vi "Read Exception Status Response.vi"(8 "error in (no error)":errorcluster, 10 "Modbus data unit in":refnum<class "Modbus Data Unit (PDU).lvclass">) -> (0 "error out":errorcluster, 2 "exception status":u8)   [LabVIEW 2018, in "SubVIs.lvlib" / "Master Function Definition.lvlib"]
doc: "Decodes the response generated by the read exception status function."
uses:
  Master Function Definition.lvlib
  Modbus Data Unit (PDU).lvclass
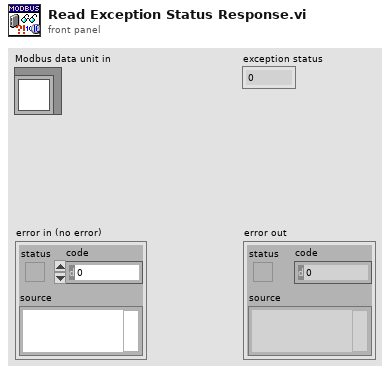
[diagram p1: front panel]
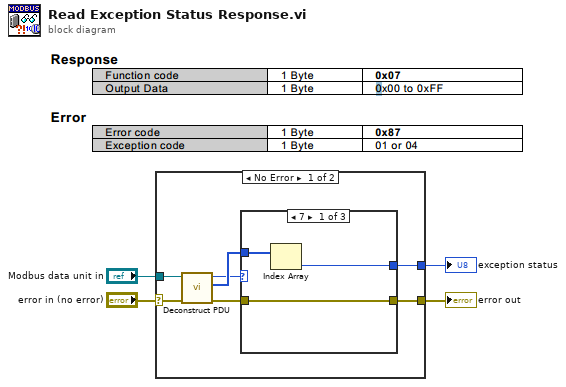
[diagram p0: block diagram]
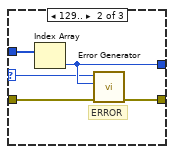
[diagram p2: hidden frame]
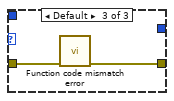
[diagram p3: hidden frame]
diagram:
  n1 = case shown="No Error" "error in (no error)" {
    selector: "error in (no error)" -> [w10 w22]
    tunnel: [w11 w22] -> w3
    tunnel: "Modbus data unit in" -> [w8 _]
    tunnel: [w6 _] -> w1
    frame No Error {
      n2 = call "Deconstruct PDU.vi"("error in (no error)"=w10, "Modbus data unit in"=w8) -> ("error out"=w7:errorcluster, "data"=w9:u8[], "function"=w5:u8)  [unwired: 7 in]
      n3 = case shown="7" w5 {
        selector: w5 -> [_ w15 _]
        tunnel: w7 -> [w13 w17 w21]
        tunnel: w9 -> [w14 w19 _]
        tunnel: [w13 w18 w20] -> w11
        tunnel: [w12 w16 _] -> w6
        frame 7 {
          n4 = Index Array(array=w14) -> (element=w12:u8)  [unwired: 1 in]
        }
        frame 129.. {
          # "ERROR"
          n5 = Index Array(array=w19) -> (element=w16:u8)  [unwired: 1 in]
          n6 = call "Error Generator.vi"("error in (no error)"=w17, "data return (error code)"=w16, "function return"=w15) -> ("error out"=w18:errorcluster)  [unwired: 8 in]
        }
        frame Default {
          n7 = call "Function code mismatch error.vi"("error in (no error)"=w21) -> ("error out"=w20:errorcluster)  [unwired: 10 in]
        }
      }
    }
    frame Error {
    }
  }
  "error out" <- w3
  "exception status" <- w1
